vi "Panel.vi"(11 "ElementEditorPanel in":refnum<class "ElementEditorPanel.lvclass">) -> ()   [LabVIEW 2020, in "VolatusGUIControls.lvlib" / "ElementEditorPanel.lvclass"]
uses:
  ElementEditorPanel.lvclass
  C:/dev/lv20CE/relink/lv-oopanel/OOPanel/Panel/Panel.lvclass
  lv-oopanel/OOPanel/Panel/Basic UI State.ctl
  ElementEditorPanel.lvclass/ElementEditorPanel.ctl
  lv-oopanel/OOPanel/Panel/Panel.lvclass
  lv-oopanel/OOPanel/OOPanel.lvlib
panel:
  # "No custom editor is available for this control."
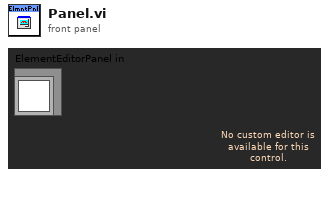
[diagram p1: front panel]
types:
  T1 = typedef "OOPanel.lvlib/Panel.lvclass/Basic UI State.ctl" = enum16{"Init", "Run", "Close"}
  T2 = typedef "OOPanel.lvlib/Panel.lvclass/Panel Events.ctl" = cluster{"Visbility":refnum<user-event>, "Close":refnum<user-event>}
  T3 = typedef "OOPanel.lvlib/Visibility State.ctl" = enum16{"Idle", "Closed", "Hidden", "Visible", "Subpanel", "Hidden Subpanel"}
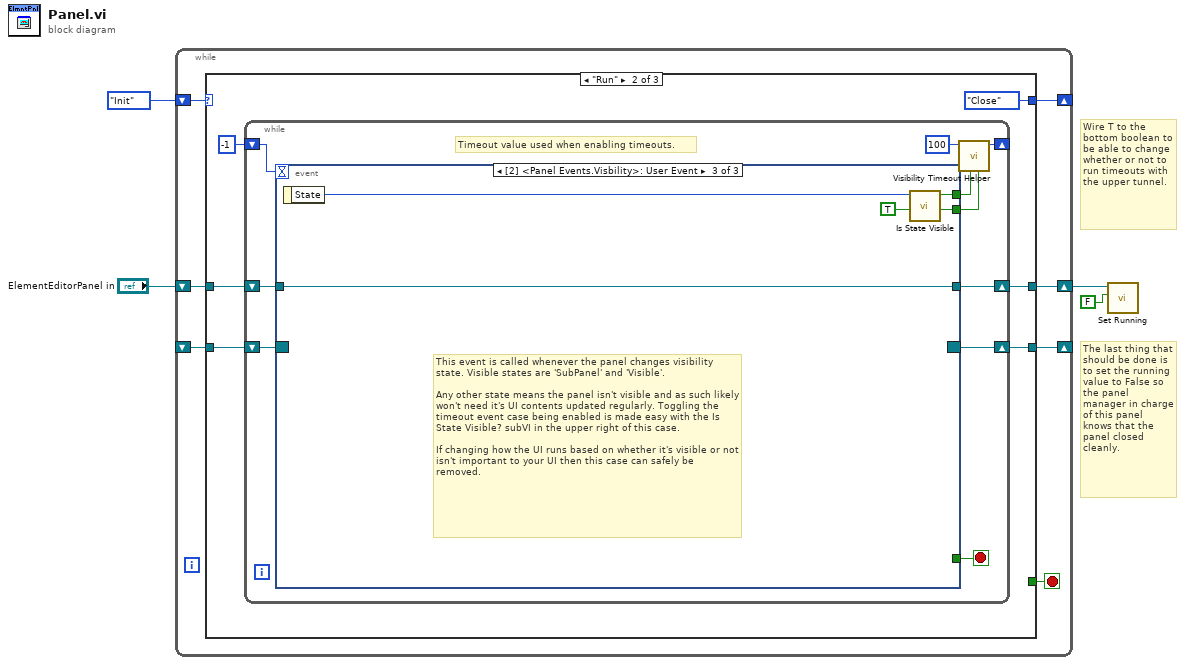
[diagram p0: block diagram]
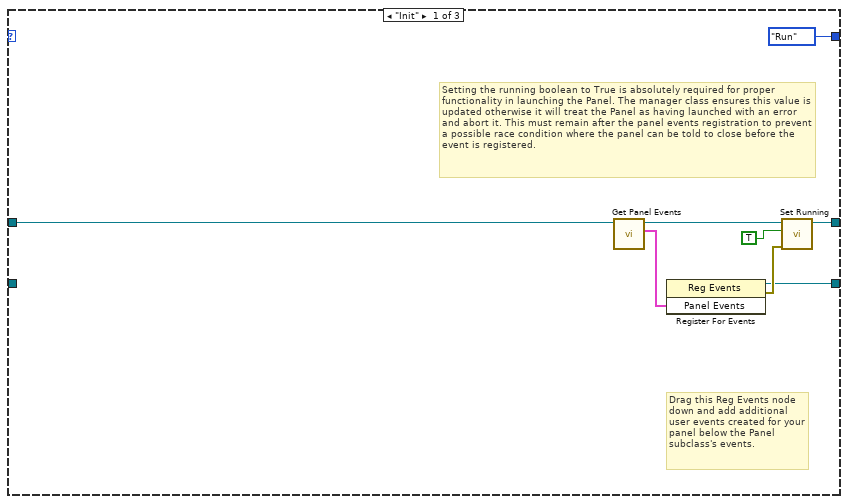
[diagram p2: hidden frame]
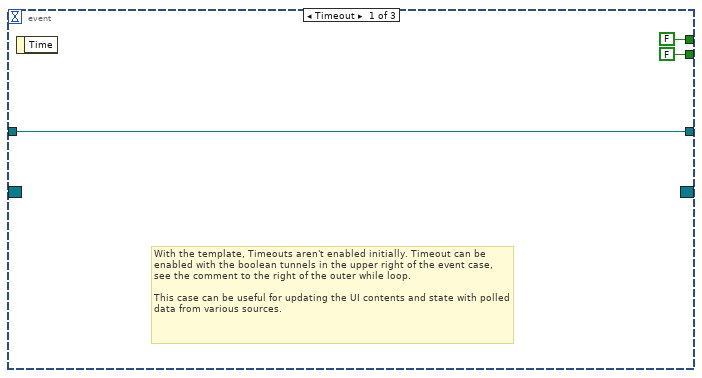
[diagram p3: hidden frame]
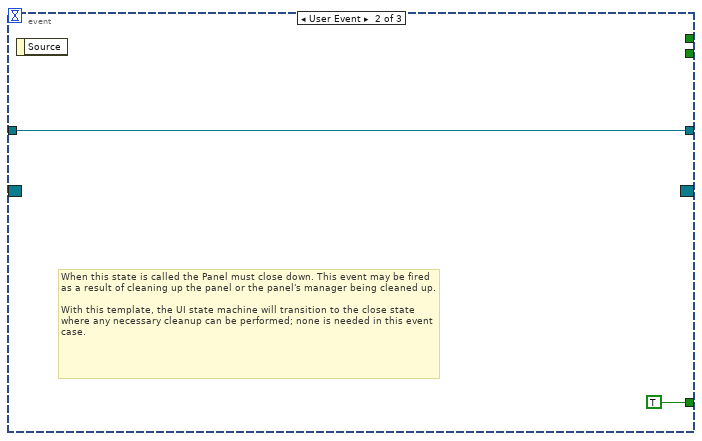
[diagram p4: hidden frame]
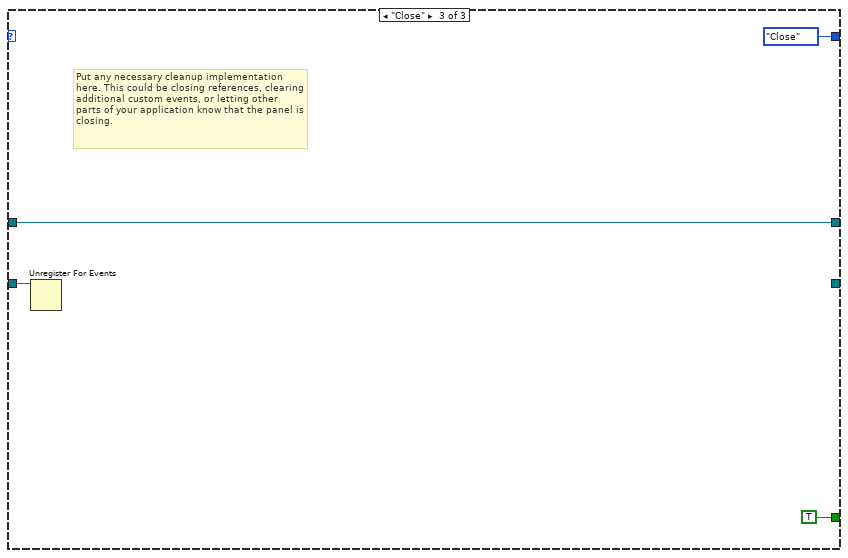
[diagram p5: hidden frame]
diagram:
  # "The last thing that should be done is to set the running value to False so the panel manager in charge of this panel knows that the panel closed cleanly."
  # "Wire T to the bottom boolean to be able to change whether or not to run timeouts with the upper tunnel."
  n1 = while {
    shift-right: [w10] -> _
    shift-left: _ -> [w11]
    shift-right: [w8] -> _
    shift-left: Basic_UI_State."Init" ("Basic UI State") -> [w9]
    shift-right: [w6] -> w4
    shift-left: "ElementEditorPanel in" -> [w5]
    stop <- w7 stop-if-true
    n2 = case shown="\"Run\"" w9 {
      tunnel: w11 -> [_ w25 w46]
      tunnel: [w16 w23 _] -> w10
      tunnel: [Basic_UI_State."Run" ("Basic UI State") Basic_UI_State."Close" ("Basic UI State") Basic_UI_State."Close" ("Basic UI State")] -> w8
      tunnel: [_ _ TRUE] -> w7
      tunnel: [w15 w20 w45] -> w6
      tunnel: w5 -> [w14 w21 w45]
      frame "Init" {
        # "Setting the running boolean to True is absolutely required for proper functionality in launching the Panel. The manager class ensures this value is updated otherwise it will treat the Panel as having launched with an error and abort it. This must remain after the panel events registration to prevent a possible race condition where the panel can be told to close before the event is registered."
        # "Drag this Reg Events node down and add additional user events created for your panel below the Panel subclass's events."
        n3 = call "Get Panel Events.vi"("Panel in"=w14) -> ("Panel Events"=w12:T2, "Panel out"=w13:refnum<class "ElementEditorPanel.lvclass">)  [unwired: 8 in, 1 out]
        n4 = register-events(w12) -> (reference out=w16:refnum<event-registration>, error out=w18:errorcluster)  [unwired: 2 in]
        n5 = call "Set Running.vi"("error in (no error)"=w18, "Running"=TRUE, "Panel in"=w13) -> ("Panel out"=w15:refnum<class "ElementEditorPanel.lvclass">)  [unwired: 7 in, 1 out]
      }
      frame "Run" {
        n6 = while {
          shift-right: [w31] -> w23
          shift-left: w25 -> [w32]
          shift-right: [w34] -> _
          shift-left: -1 ("Timeout") -> [w33]
          shift-right: [w26] -> w20
          shift-left: w21 -> [w27]
          stop <- w28 stop-if-true
          # "Timeout value used when enabling timeouts."
          n7 = event shown="[2] <Panel Events.Visbility>: User Event" {
            selector: w32 -> [_ _ _]
            dyn-events: [_ _ _] -> w31
            timeout: w33 -> [_ _ _]
            tunnel: [FALSE _ w43] -> w30
            tunnel: [FALSE _ TRUE] -> w29
            tunnel: [_ TRUE _] -> w28
            tunnel: w27 -> [w36 w39 w41]
            tunnel: [w36 w39 w41] -> w26
            event Timeout {
              # "With the template, Timeouts aren't enabled initially. Timeout can be enabled with the boolean tunnels in the upper right of the event case, see the comment to the right of the outer while loop.\n\nThis case can be useful for updating the UI contents and state with polled data from various sources."
              n8 = event-data() -> ()  [unwired: 1 in, 1 out]
            }
            event User Event {
              # "When this state is called the Panel must close down. This event may be fired as a result of cleaning up the panel or the panel's manager being cleaned up.\n\nWith this template, the UI state machine will transition to the close state where any necessary cleanup can be performed; none is needed in this event case."
              n9 = event-data() -> ()  [unwired: 1 in, 1 out]
            }
            event User Event {
              # "This event is called whenever the panel changes visibility state. Visible states are 'SubPanel' and 'Visible'.\n\nAny other state means the panel isn't visible and as such likely won't need it's UI contents updated regularly. Toggling the timeout event case being enabled is made easy with the Is State Visible? subVI in the upper right of this case.\n\nIf changing how the UI runs based on whether it's visible or not isn't important to your UI then this case can safely be removed."
              n10 = event-data() -> ("State"=w44:T3)  [unwired: 1 in]
              n11 = call "Is State Visible.vi"("Visibility"=w44) -> ("Visible"=w43:bool)  [unwired: 10 in]
            }
          }
          n12 = call "Visibility Timeout Helper.vi"("Update?"=w29, "Use Timeout?"=w30, "Visible Timeout mS"=100) -> ("Timeout"=w34:i32)  [unwired: 8 in]
        }
      }
      frame "Close" {
        # "Put any necessary cleanup implementation here. This could be closing references, clearing additional custom events, or letting other parts of your application know that the panel is closing."
        n13 = Unregister For Events(event registration refnum=w46) -> ()  [unwired: 1 in, 1 out]
      }
    }
  }
  n14 = call "Set Running.vi"("Running"=FALSE, "Panel in"=w4) -> ()  [unwired: 8 in, 2 out]
